vi "getParameters.vi"(8 "error in (no error)":errorcluster, 11 "IEventPacket in":refnum<class "IEventPacket.lvclass">) -> (0 "error out":errorcluster, 2 "Parameters out":refnum<class "IDict.lvclass">, 3 "IEventPacket out":refnum<class "IEventPacket.lvclass">)   [LabVIEW 2022 SP3, in "openDAQ.lvlib" / "IBaseObject.lvlib" / "IPacket.lvlib" / "IEventPacket.lvlib" / "IEventPacket.lvclass"]
uses:
  <instrlib>/openDAQ/Public/Classes/IEventPacket/IEventPacket.lvclass
  C:/Program Files (x86)/National Instruments/LabVIEW 2022/instr.lib/openDAQ/Public/Classes/IBaseObject/IBaseObject.lvclass
  <instrlib>/openDAQ/Public/Classes/daqCoreTypes/IDict/IDict.lvclass
  <instrlib>/openDAQ/Public/Classes/IBaseObject/IBaseObject.lvclass/IBaseObject.ctl
  <instrlib>/openDAQ/Public/Classes/IBaseObject/Accessor/Read reference.vi
  <instrlib>/openDAQ/Public/Classes/IBaseObject/Accessor/Write reference.vi
  <instrlib>/openDAQ/Binaries/Windows/x86/copendaq32.dll
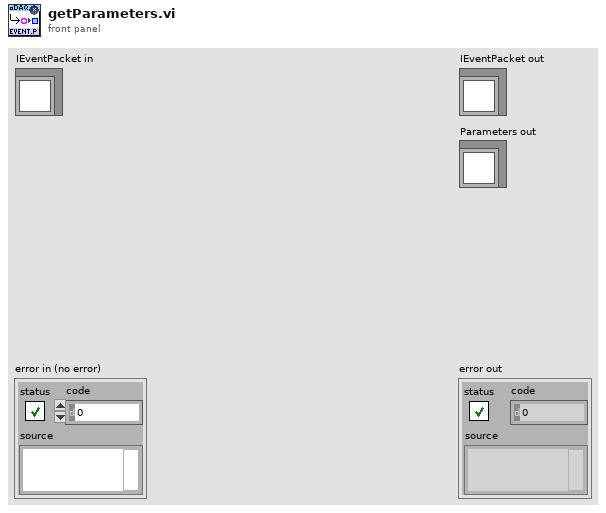
[diagram p1: front panel]
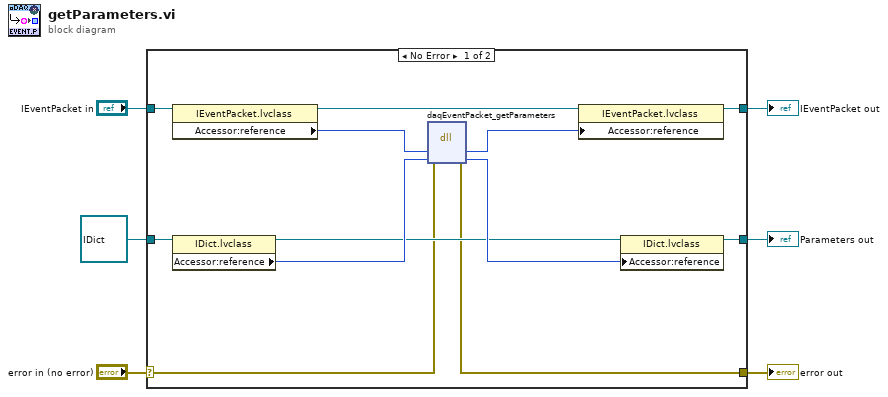
[diagram p0: block diagram]
diagram:
  n1 = case shown="No Error" "error in (no error)" {
    selector: "error in (no error)" -> [w10 w21]
    tunnel: [w8 w21] -> w5
    tunnel: [w11 w20] -> w3
    tunnel: "IEventPacket in" -> [w18 w20]
    tunnel: [w7 w19] -> w1
    tunnel: refnum<class "IDict.lvclass"> refnum ("openDAQ.lvlib:daqCoreTypes.lvlib:IDict.lvclass") -> [w9 w19]
    frame No Error {
      n2 = property class="IEventPacket.lvclass"(reference=w18) -> (reference out=w12:refnum<class "IEventPacket.lvclass">, "Accessor:reference"=w17:i64)  [unwired: 1 in, 1 out]
      n3 = property class="IDict.lvclass"(reference=w9) -> (reference out=w13:refnum<class "IDict.lvclass">, "Accessor:reference"=w15:i64)  [unwired: 1 in, 1 out]
      n4 = dll-call lib="C:/Program Files (x86)/National Instruments/LabVIEW 2022/instr.lib/openDAQ/Binaries/Windows/x86/copendaq*.*" fn="daqEventPacket_getParameters"(error in=w10, "eventPacket"=w17, "parameters"=w15) -> (error out=w8:errorcluster, "eventPacket"=w16:i64, "parameters"=w14:i64)  [unwired: 3 in, 1 out]
      n5 = property class="IEventPacket.lvclass"(reference=w12, "Accessor:reference"=w16) -> (reference out=w11:refnum<class "IEventPacket.lvclass">)  [unwired: 1 in, 1 out]
      n6 = property class="IDict.lvclass"(reference=w13, "Accessor:reference"=w14) -> (reference out=w7:refnum<class "IDict.lvclass">)  [unwired: 1 in, 1 out]
    }
    frame Error {
    }
  }
  "error out" <- w5
  "IEventPacket out" <- w3
  "Parameters out" <- w1
